vi "CreateSweep.vi"(6 "Sweeps":dbl, 9 "Number Points":dbl, 10 "Minimum Voltage":dbl, 11 "Maxiumum Voltage":dbl) -> (2 "XY pairs":cluster{"x":timestamp, "y":dbl}[](array[cluster]), 3 "Waveform":waveform(dbl))   [LabVIEW 2020]
uses:
  <vilib>/Waveform/WDTOps.llb/WDT Waveform to XY Pairs DBL.vi
  <vilib>/measure/NI_MABase.lvlib
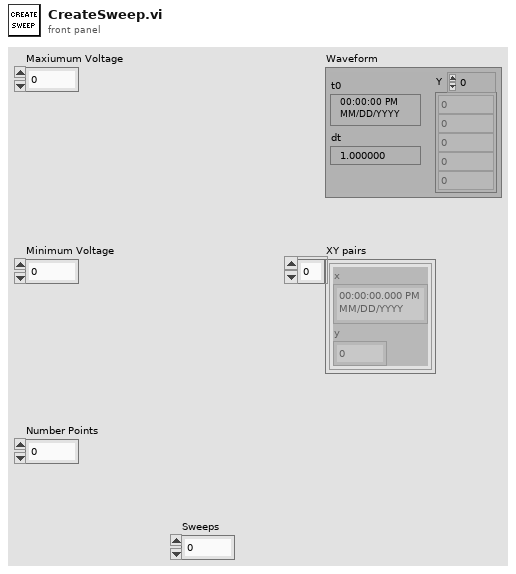
[diagram p1: front panel]
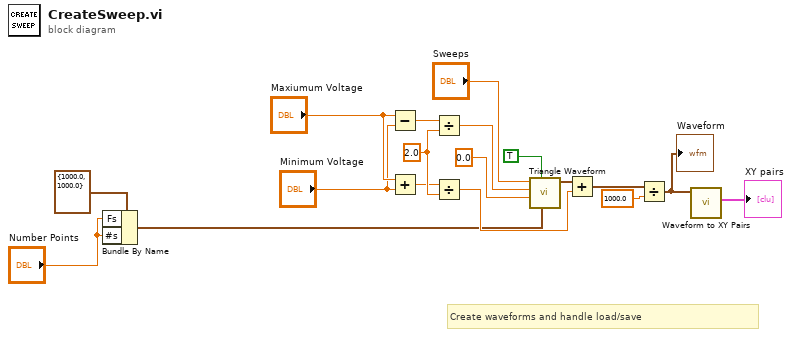
[diagram p0: block diagram]
diagram:
  w14 = 2.0 ("y")
  # "Create waveforms and handle load/save"
  n1 = Bundle By Name(cluster=cluster{"Fs":dbl, "#s":dbl} {"Fs"=1000.0, "#s"=1000.0} ("sampling info"), "Fs"="Number Points", "#s"="Number Points") -> (w2:cluster{"Fs":dbl, "#s":dbl})
  n2 = Subtract(x="Maxiumum Voltage", y="Minimum Voltage") -> (x-y=w11:dbl)
  n3 = Add(x="Maxiumum Voltage", y="Minimum Voltage") -> (x+y=w5:dbl)
  n4 = Divide(x=w11, y=w14) -> (x/y=w9:dbl)
  n5 = Divide(x=w5, y=w14) -> (x/y=w4:dbl)
  n6 = call <vilib>:"Triangle Waveform.vi"("sampling info"=w2, "reset signal"=TRUE, "phase"=0.0, "amplitude"=w9, "frequency"="Sweeps") -> ("signal out"=w8:waveform(dbl))  [unwired: 5 in, 1 out]
  n7 = Add(x=w8, y=w4) -> (x+y=w3:waveform(dbl))
  n8 = Divide(x=w3, y=1000.0) -> (x/y=w18:waveform(dbl))
  "Waveform" <- w18
  n9 = call-poly <vilib>:"Waveform to XY Pairs.vi"("waveform in"=w18) -> ("XY pairs"=→"XY pairs":cluster{"x":timestamp, "y":dbl}[])  [unwired: 8 in, 2 out]
